vi "Get_sw.vi"(8 "error in (no error)":errorcluster, 11 "Lifter_motor in":refnum<class "Lifter_motor.lvclass">) -> (0 "error out":errorcluster, 2 "Switch Hex":dbl, 3 "Lifter_motor out":refnum<class "Lifter_motor.lvclass">)   [LabVIEW 2019, in "Lifter_motor.lvclass"]
uses:
  Lifter_motor.lvclass
  Lifter_motor.lvclass/Lifter_motor.ctl
  TCP Class/LifterTCP.lvclass
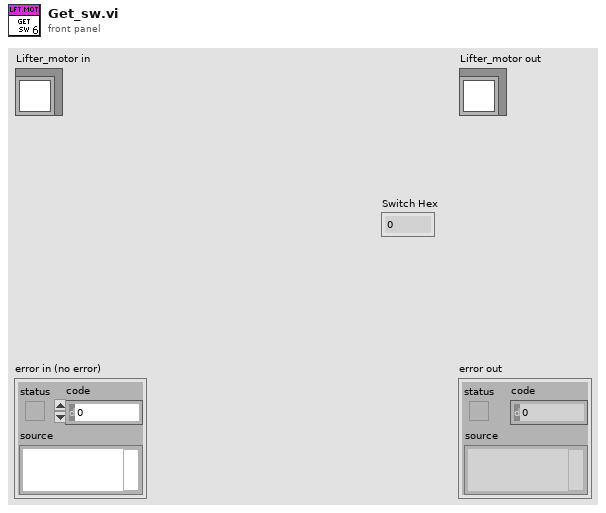
[diagram p1: front panel]
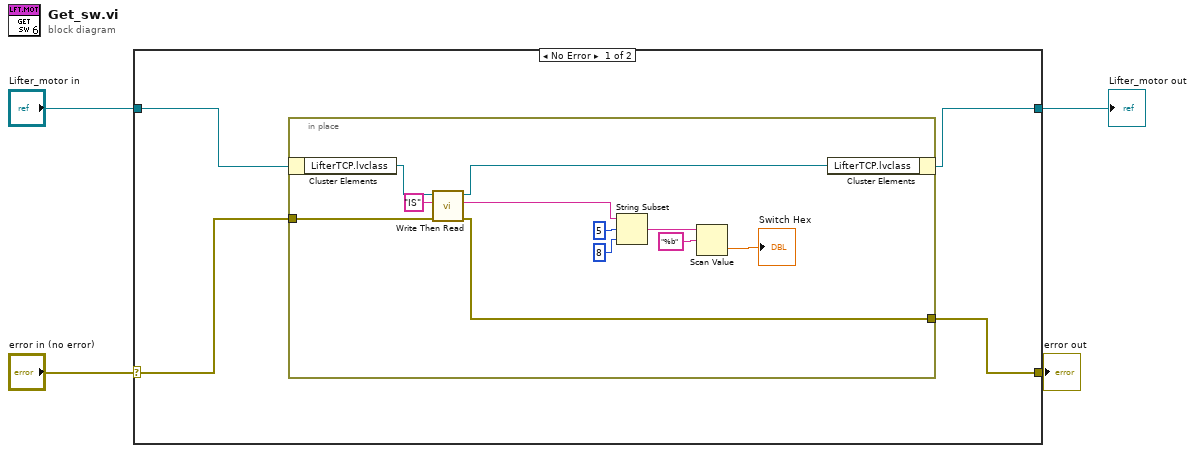
[diagram p0: block diagram]
diagram:
  n1 = case shown="No Error" "error in (no error)" {
    selector: "error in (no error)" -> [w6 w21]
    tunnel: [w5 w21] -> w3
    tunnel: [w7 w20] -> w1
    tunnel: "Lifter_motor in" -> [w8 w20]
    frame No Error {
      n2 = in-place {
        in-place-border: w6 -> [w18]
        in-place-border: [w10] -> w5
        n3 = in-place-cluster #1(w8) -> ("LifterTCP.lvclass"=w19:refnum<class "LifterTCP.lvclass">)
        n4 = call "Write Then Read.vi"("error in (no error)"=w18, "Parameter 1"="IS", "LifterTCP in"=w19) -> ("error out"=w10:errorcluster, "Read Data"=w12:string, "LifterTCP out"=w11:refnum<class "LifterTCP.lvclass">)  [unwired: 6 in]
        n5 = String Subset(string=w12, offset (0)=5, length (rest)=8 ("length (rest)")) -> (substring=w17:string)
        n6 = Scan Value(string=w17, format string="%b") -> (value=→"Switch Hex":dbl)  [unwired: 1 in, 1 out]
        n7 = in-place-cluster #1("LifterTCP.lvclass"=w11) -> (w7:refnum<class "Lifter_motor.lvclass">)
      }
    }
    frame Error {
    }
  }
  "error out" <- w3
  "Lifter_motor out" <- w1
